vi "GaAsP_GaAs_SL.vi"(2 "Debug Mode":bool, 3 "Elapsed Time(s)":dbl, 4 "State":enum16{"Edit", "Start", "Run", "End", "Idle"}(ring), 5 "Argument List In":string[](array[string])) -> (0 "Status Out":string, 1 "Argument List Out":string[](array[string]))   [LabVIEW 2011]
panel:
  in  "As flow1 (sccm)":dbl
  out "tphase(s)":dbl[](array[numeric])
  out "nstep":dbl
  out "phase":i32
  out "done":bool
  in  "t1wait (s)":dbl
  in  "t1 flow (s)":dbl
  in  "P flow1 (sccm)":dbl
  in  "nPeriods":dbl
  out "tTotal(s)":dbl
  out "tPeriod(s)":dbl
  in  "t2 wait (s)":dbl
  in  "t2 flow (s)":dbl
  in  "As flow2 (sccm)":dbl
  in  "Cancel":bool
  in  "OK":bool
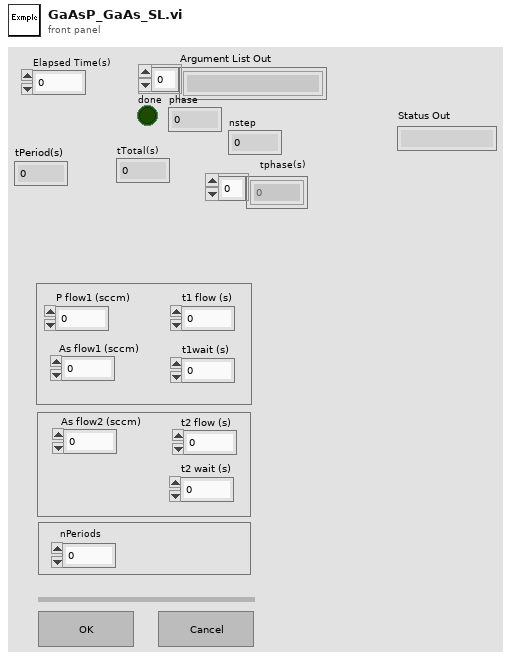
[diagram p1: front panel]
types:
  T1 = enum16{"Discrete", "Continuous", "Instantaneous"}
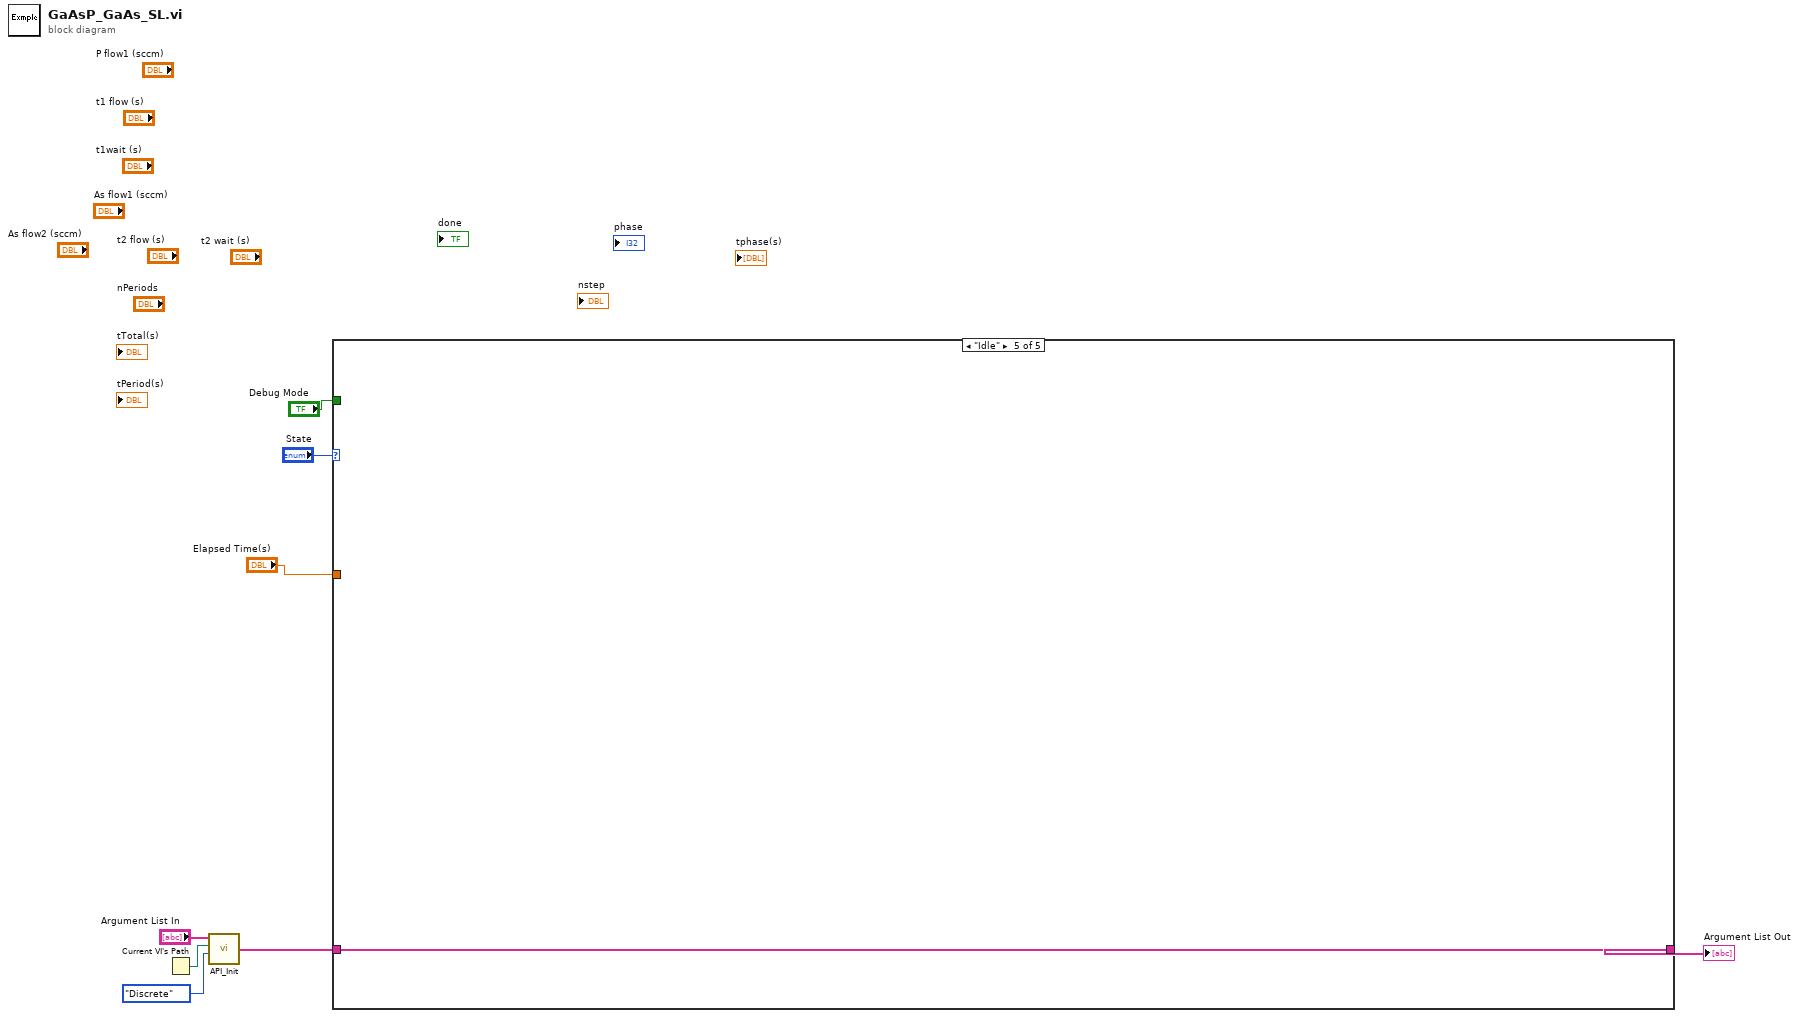
[diagram p0: block diagram]
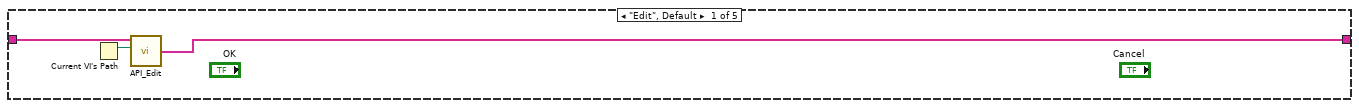
[diagram p2: hidden frame]
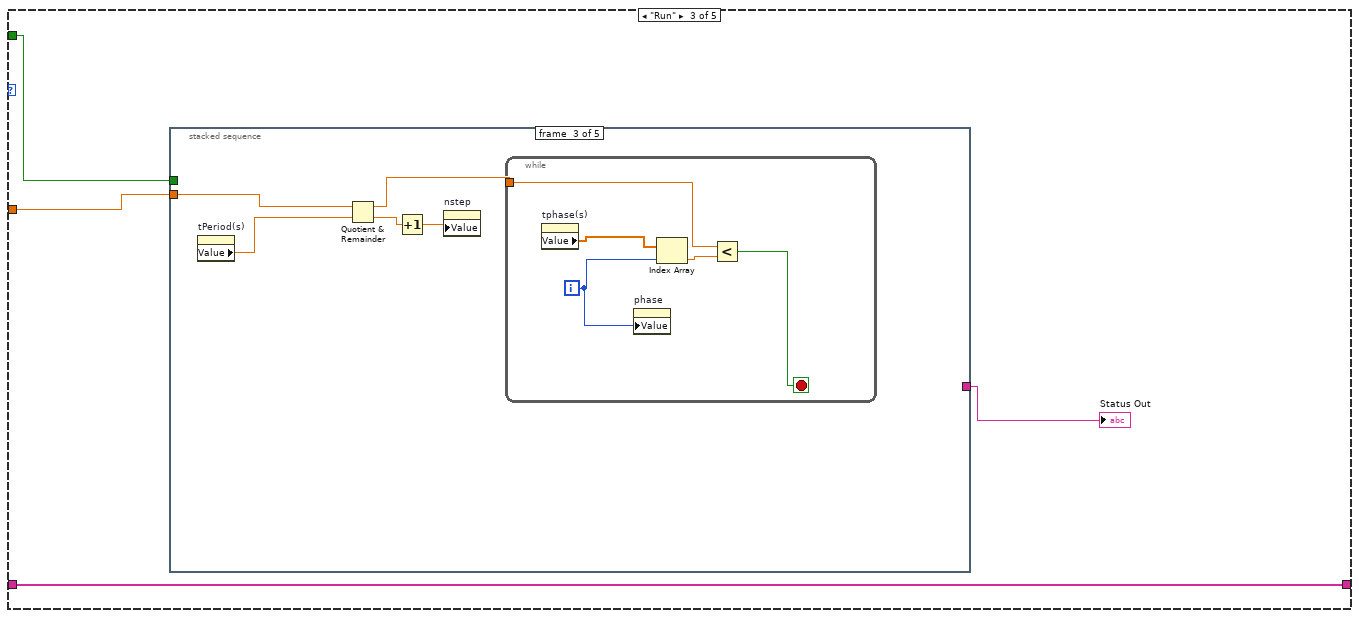
[diagram p4: hidden frame]
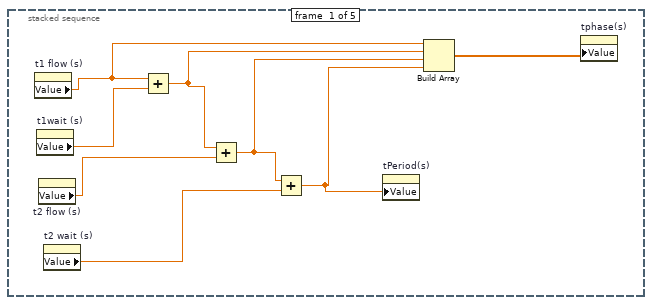
[diagram p5: hidden frame]
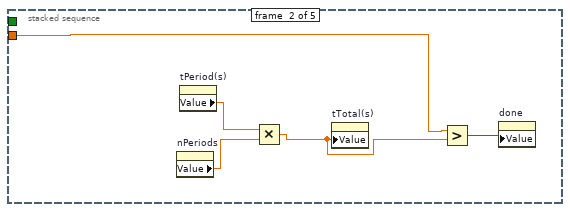
[diagram p6: hidden frame]
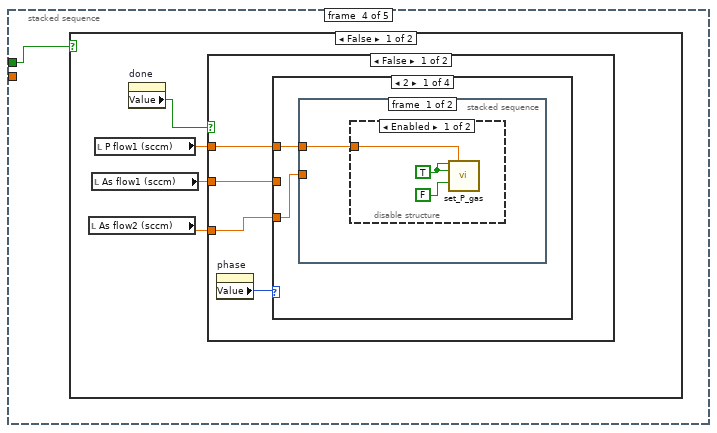
[diagram p7: hidden frame]
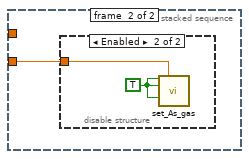
[diagram p9: hidden frame]
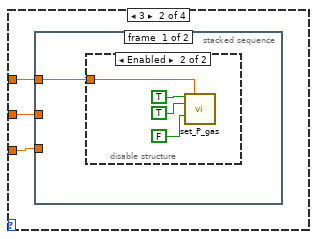
[diagram p11: hidden frame]
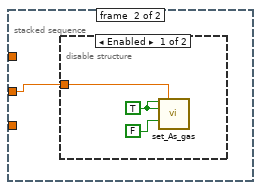
[diagram p13: hidden frame]
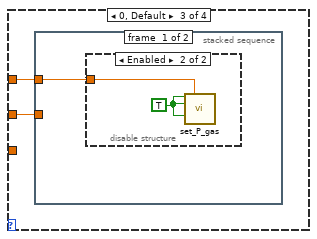
[diagram p15: hidden frame]
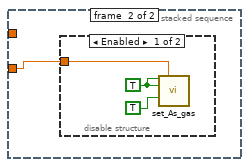
[diagram p17: hidden frame]
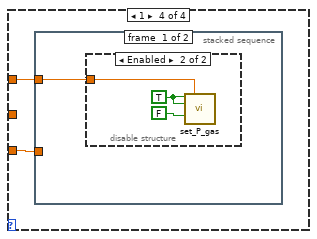
[diagram p19: hidden frame]
diagram:
  n1 = Current VI's Path() -> (path=w5:path)
  n2 = call "API_Init.vi"("API Mode"=T1."Discrete", "VI Path"=w5, "Argument List In"="Argument List In") -> ("Argument List Out"=w6:string[])  [unwired: 1 in]
  n3 = case shown="\"Idle\"" "State" {
    tunnel: [w9 w12 w16 w136 w137] -> w2
    tunnel: w6 -> [w11 w12 w16 w136 w137]
    tunnel: "Debug Mode" -> [_ _ w14 _ _]
    tunnel: "Elapsed Time(s)" -> [_ _ w15 _ _]
    frame "Edit", Default {
      n4 = Current VI's Path() -> (path=w10:path)
      n5 = call "API_Edit.vi"("VI Path"=w10, "Argument List In"=w11) -> ("Argument List Out"=w9:string[])  [unwired: 2 in]
    }
    frame "Start" {
    }
    frame "Run" {
      n6 = stacked-sequence {
        tunnel: w15 -> [_ w27 w34 _ _]
        tunnel: w14 -> [_ _ _ w40 _]
        tunnel: [_ _ _ _ w99] -> w13
        frame #0 {
          n7 = property on="t1 flow (s)" class="DigNum (strict)"() -> ("Value"=w23:dbl)  [unwired: 2 in, 2 out]
          n8 = property on="t1wait (s)" class="DigNum (strict)"() -> ("Value"=w24:dbl)  [unwired: 2 in, 2 out]
          n9 = property on="t2 flow (s)" class="DigNum (strict)"() -> ("Value"=w21:dbl)  [unwired: 2 in, 2 out]
          n10 = property on="t2 wait (s)" class="DigNum (strict)"() -> ("Value"=w20:dbl)  [unwired: 2 in, 2 out]
          n11 = Add(x=w23, y=w24) -> (x+y=w22:dbl)
          n12 = Add(x=w22, y=w21) -> (x+y=w19:dbl)
          n13 = Add(x=w19, y=w20) -> (x+y=w18:dbl)
          n14 = property on="tPeriod(s)" class="DigNum (strict)"("Value"=w18) -> ()  [unwired: 2 in, 2 out]
          n15 = Build Array(w23, w22, w19, w18) -> (w17:dbl[])
          n16 = property on="tphase(s)" class="Arr (strict)"("Value"=w17) -> ()  [unwired: 2 in, 2 out]
        }
        frame #1 {
          n17 = property on="nPeriods" class="DigNum (strict)"() -> ("Value"=w28:dbl)  [unwired: 2 in, 2 out]
          n18 = property on="tPeriod(s)" class="DigNum (strict)"() -> ("Value"=w29:dbl)  [unwired: 2 in, 2 out]
          n19 = Multiply(x=w29, y=w28) -> (x*y=w26:dbl)
          n20 = property on="tTotal(s)" class="DigNum (strict)"("Value"=w26) -> ()  [unwired: 2 in, 2 out]
          n21 = Greater?(x=w27, y=w26) -> (0:w25:bool)
          n22 = property on="done" class="Bool (strict)"("Value"=w25) -> ()  [unwired: 2 in, 2 out]
        }
        frame #2 {
          n23 = property on="tPeriod(s)" class="DigNum (strict)"() -> ("Value"=w33:dbl)  [unwired: 2 in, 2 out]
          n24 = Quotient & Remainder(x=w34, y=w33) -> (x-y*floor(x/y)=w32:dbl, floor(x/y)=w31:dbl)
          n25 = Increment(x=w31) -> (x+1=w30:dbl)
          n26 = property on="nstep" class="DigNum (strict)"("Value"=w30) -> ()  [unwired: 2 in, 2 out]
          n27 = while {
            tunnel: w32 -> [w38]
            i -> [w36]
            stop <- w35 stop-if-true
            n28 = property on="tphase(s)" class="Arr (strict)"() -> ("Value"=w39:dbl[])  [unwired: 2 in, 2 out]
            n29 = property on="phase" class="DigNum (strict)"("Value"=w36) -> ()  [unwired: 2 in, 2 out]
            n30 = Index Array(array=w39, index=w36) -> (element=w37:dbl)
            n31 = Less?(x=w38, y=w37) -> (x < y?=w35:bool)
          }
        }
        frame #3 {
          n32 = case shown="False" w40 {
            frame False {
              n33 = local read "As flow2 (sccm)"() -> (w44:dbl)
              n34 = local read "As flow1 (sccm)"() -> (w41:dbl)
              n35 = local read "P flow1 (sccm)"() -> (w43:dbl)
              n36 = property on="done" class="Bool (strict)"() -> ("Value"=w42:bool)  [unwired: 2 in, 2 out]
              n37 = case shown="False" w42 {
                tunnel: w44 -> [w48 w89]
                tunnel: w43 -> [w47 w90]
                tunnel: w41 -> [w45 _]
                frame False {
                  n38 = property on="phase" class="DigNum (strict)"() -> ("Value"=w46:i32)  [unwired: 2 in, 2 out]
                  n39 = case shown="2" w46 {
                    tunnel: w47 -> [w50 w60 w71 w80]
                    tunnel: w48 -> [w49 w59 _ w79]
                    tunnel: w45 -> [_ w58 w70 _]
                    frame 2 {
                      n40 = stacked-sequence {
                        tunnel: w50 -> [w51 _]
                        tunnel: w49 -> [_ w55]
                        frame #0 {
                          n41 = disable-structure shown="Enabled" {
                            disable-tunnel: w51 -> [w52 _]
                            frame Enabled {
                              w54 = TRUE ("Ga Active")
                              n42 = call "set_P_gas.vi"("P_Gas Active"=w54, "P_Gas Flow"=w52, "P_Gas In"=w54, "P_Gas Run"=FALSE ("Al Run")) -> ()  [unwired: 12 in]
                            }
                            frame Disabled {
                            }
                          }
                        }
                        frame #1 {
                          n43 = disable-structure shown="Enabled" {
                            disable-tunnel: w55 -> [_ w57]
                            frame Disabled {
                            }
                            frame Enabled {
                              w56 = TRUE ("Ga Active")
                              n44 = call "set_As_gas.vi"("As_Gas Active"=w56, "As_Gas Flow"=w57, "As_Gas In"=w56, "As_Gas Run"=w56) -> ()  [unwired: 12 in]
                            }
                          }
                        }
                      }
                    }
                    frame 3 {
                      n45 = stacked-sequence {
                        tunnel: w60 -> [w61 _]
                        tunnel: w59 -> [_ _]
                        tunnel: w58 -> [_ w66]
                        frame #0 {
                          n46 = disable-structure shown="Enabled" {
                            disable-tunnel: w61 -> [_ w62]
                            frame Disabled {
                            }
                            frame Enabled {
                              n47 = call "set_P_gas.vi"("P_Gas Active"=TRUE ("Al Active"), "P_Gas Flow"=w62, "P_Gas In"=TRUE ("Al Bubbler"), "P_Gas Run"=FALSE ("Al Run")) -> ()  [unwired: 12 in]
                            }
                          }
                        }
                        frame #1 {
                          n48 = disable-structure shown="Enabled" {
                            disable-tunnel: w66 -> [w67 _]
                            frame Enabled {
                              w68 = TRUE ("Ga Active")
                              n49 = call "set_As_gas.vi"("As_Gas Active"=w68, "As_Gas Flow"=w67, "As_Gas In"=w68, "As_Gas Run"=FALSE ("Ga Run")) -> ()  [unwired: 12 in]
                            }
                            frame Disabled {
                            }
                          }
                        }
                      }
                    }
                    frame 0, Default {
                      n50 = stacked-sequence {
                        tunnel: w71 -> [w72 _]
                        tunnel: w70 -> [_ w75]
                        frame #0 {
                          n51 = disable-structure shown="Enabled" {
                            disable-tunnel: w72 -> [_ w74]
                            frame Disabled {
                            }
                            frame Enabled {
                              w73 = TRUE ("Al Active")
                              n52 = call "set_P_gas.vi"("P_Gas Active"=w73, "P_Gas Flow"=w74, "P_Gas In"=w73, "P_Gas Run"=w73) -> ()  [unwired: 12 in]
                            }
                          }
                        }
                        frame #1 {
                          n53 = disable-structure shown="Enabled" {
                            disable-tunnel: w75 -> [w76 _]
                            frame Enabled {
                              w77 = TRUE ("Ga Active")
                              n54 = call "set_As_gas.vi"("As_Gas Active"=w77, "As_Gas Flow"=w76, "As_Gas In"=w77, "As_Gas Run"=TRUE ("Ga Run")) -> ()  [unwired: 12 in]
                            }
                            frame Disabled {
                            }
                          }
                        }
                      }
                    }
                    frame 1 {
                      n55 = stacked-sequence {
                        tunnel: w79 -> [_ w85]
                        tunnel: w80 -> [w81 _]
                        frame #0 {
                          n56 = disable-structure shown="Enabled" {
                            disable-tunnel: w81 -> [_ w83]
                            frame Disabled {
                            }
                            frame Enabled {
                              w82 = TRUE ("Al Bubbler")
                              n57 = call "set_P_gas.vi"("P_Gas Active"=w82, "P_Gas Flow"=w83, "P_Gas In"=w82, "P_Gas Run"=FALSE ("Al Run")) -> ()  [unwired: 12 in]
                            }
                          }
                        }
                        frame #1 {
                          n58 = disable-structure shown="Disabled" {
                            disable-tunnel: w85 -> [w86 _]
                            frame Enabled {
                              w87 = TRUE ("Ga Active")
                              n59 = call "set_As_gas.vi"("As_Gas Active"=w87, "As_Gas Flow"=w86, "As_Gas In"=w87, "As_Gas Run"=FALSE ("Ga Run")) -> ()  [unwired: 12 in]
                            }
                            frame Disabled {
                            }
                          }
                        }
                      }
                    }
                  }
                }
                frame True {
                  n60 = stacked-sequence {
                    tunnel: w90 -> [w91 _]
                    tunnel: w89 -> [_ w95]
                    frame #0 {
                      n61 = disable-structure shown="Enabled" {
                        disable-tunnel: w91 -> [_ w94]
                        frame Disabled {
                        }
                        frame Enabled {
                          w93 = TRUE ("Al Active")
                          n62 = call "set_P_gas.vi"("P_Gas Active"=w93, "P_Gas Flow"=w94, "P_Gas In"=w93, "P_Gas Run"=FALSE ("Al Run")) -> ()  [unwired: 12 in]
                        }
                      }
                    }
                    frame #1 {
                      n63 = disable-structure shown="Enabled" {
                        disable-tunnel: w95 -> [w96 _]
                        frame Enabled {
                          w97 = TRUE ("Ga Active")
                          n64 = call "set_As_gas.vi"("As_Gas Active"=w97, "As_Gas Flow"=w96, "As_Gas In"=w97, "As_Gas Run"=FALSE ("Ga Run")) -> ()  [unwired: 12 in]
                        }
                        frame Disabled {
                        }
                      }
                    }
                  }
                }
              }
            }
            frame True {
            }
          }
        }
        frame #4 {
          n65 = property on="done" class="Bool (strict)"() -> ("Value"=w100:bool)  [unwired: 2 in, 2 out]
          n66 = case shown="True" w100 {
            tunnel: [w101 w135] -> w99
            frame False {
              n67 = property on="phase" class="DigNum (strict)"() -> ("Value"=w108:i32)  [unwired: 2 in, 2 out]
              n68 = case shown="1" w108 {
                tunnel: [w111 "wait (GaAs)" w118 "wait (GaPAs)"] -> w107
                frame 2 {
                  n69 = local read "As flow2 (sccm)"() -> (w110:dbl)
                  n70 = Format Into String(format string="%4.2f", w110) -> (resulting string=w114:string)  [unwired: 2 in, 1 out]
                  n71 = Concatenate Strings("As(" ("string"), w114, "sccm)" ("string")) -> (w111:string)
                }
                frame 3 {
                }
                frame 0, Default {
                  n72 = local read "P flow1 (sccm)"() -> (w124:dbl)
                  n73 = local read "As flow1 (sccm)"() -> (w123:dbl)
                  n74 = Format Into String(format string="%4.1f", w124) -> (resulting string=w126:string)  [unwired: 2 in, 1 out]
                  n75 = Format Into String(format string="%4.2f", w123) -> (resulting string=w120:string)  [unwired: 2 in, 1 out]
                  n76 = Concatenate Strings("P(" ("string"), w126, "sccm)" ("string")) -> (w119:string)
                  n77 = Concatenate Strings(w119, "As(" ("string"), w120, "sccm)" ("string")) -> (w118:string)
                }
                frame 1 {
                }
              }
              n78 = property on="nstep" class="DigNum (strict)"() -> ("Value"=w109:dbl)  [unwired: 2 in, 2 out]
              n79 = Format Into String(format string="%3.0f", w109) -> (resulting string=w104:string)  [unwired: 2 in, 1 out]
              n80 = Concatenate Strings("Period " ("string"), w104) -> (w102:string)
              n81 = Concatenate Strings(w102, ", " ("string"), w107) -> (w101:string)
            }
            frame True {
              n82 = property on="nPeriods" class="DigNum (strict)"() -> ("Value"=w130:dbl)  [unwired: 2 in, 2 out]
              n83 = Format Into String(format string="%3.0f", w130) -> (resulting string=w131:string)  [unwired: 2 in, 1 out]
              n84 = Concatenate Strings("done after", w131, " periods" ("string")) -> (w135:string)
            }
          }
        }
      }
      "Status Out" <- w13
    }
    frame "End" {
    }
    frame "Idle" {
    }
  }
  "Argument List Out" <- w2
